vi "loopback cluster (in place).vi"() -> ()   [LabVIEW 2013]
uses:
  Source/Pipes/Classes/Unix Pipe Reader/Open Pipe (reader).vi
  Source/Pipes/Classes/Unix Pipe Writer/Open Pipe (writer).vi
  Source/Pipes/Classes/Unix Pipe Reader/Close Pipe (reader).vi
  Source/Pipes/Classes/Unix Pipe Writer/Close Pipe (writer).vi
  <vilib>/NI/NI Linux RT Utilities/VIs/Public/Time/Get Clock Time (timespec).vi
  <vilib>/NI/NI Linux RT Utilities/Linux RT Utilities.lvlib
  Source/Pipes/Linux RT IPC.Pipes.lvlib
  Source/Pipes/Classes/Unix Pipe Writer/Unix Pipe Writer.lvclass
  Source/Pipes/Classes/Unix Pipe Reader/Unix Pipe Reader.lvclass
panel:
  out "read iterations":i32
  out "write iterations":i32
  in  "write":bool
  out "timed out":bool
  out "stop":bool
  out "pipe already exists?":bool
  in  "stop":bool
  out "time":cluster{"sec":u64, "nsec":u64}
  out "bytes read":i32
  out "error out":errorcluster
  out "bytes written":i32
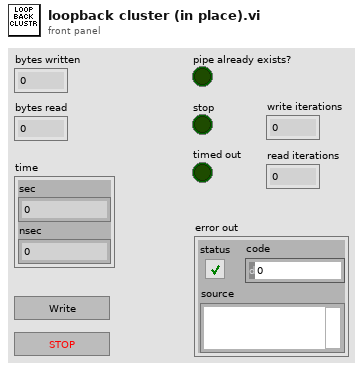
[diagram p1: front panel]
types:
  T1 = cluster{"Stop":bool, "Time":cluster{"sec":u64, "nsec":u64}}
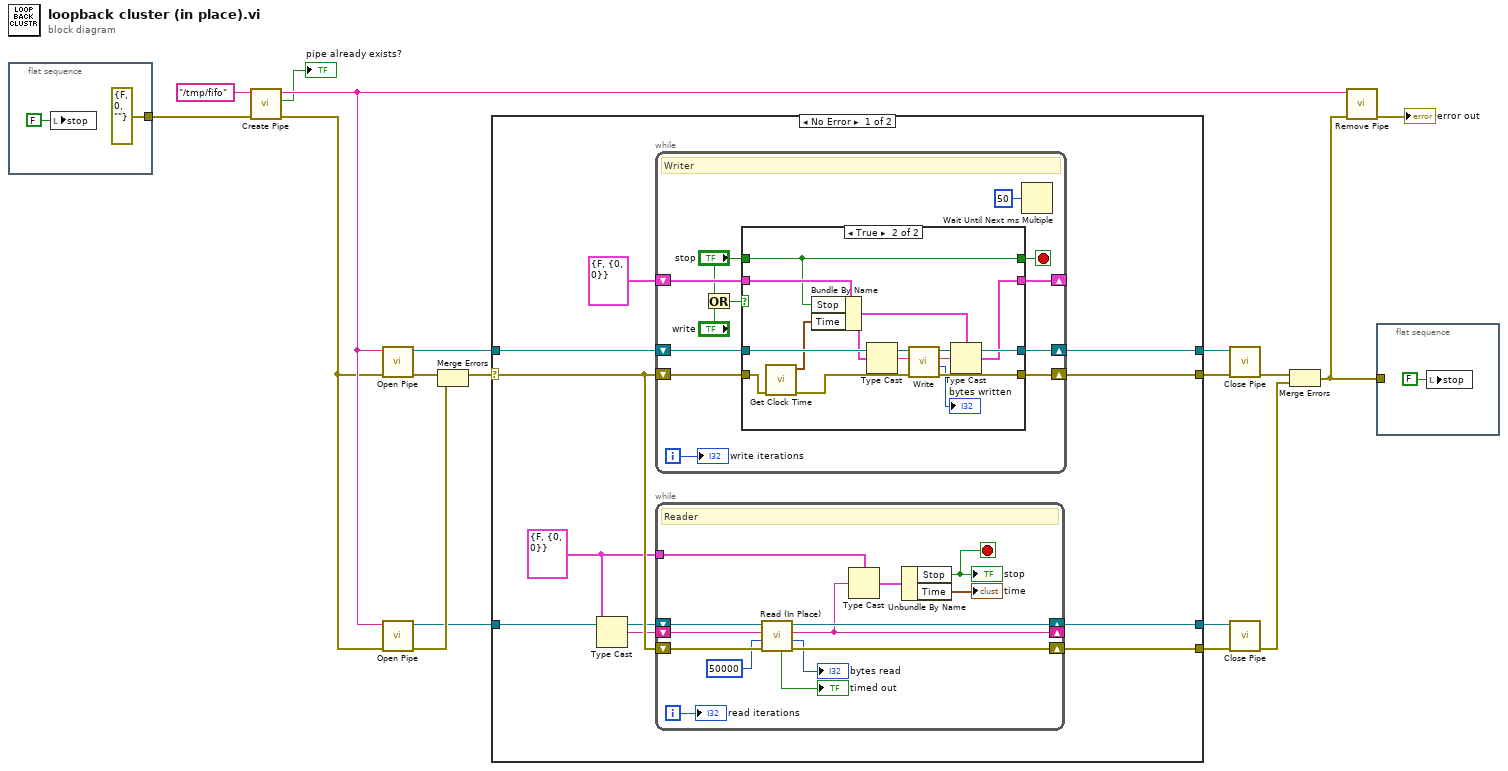
[diagram p0: block diagram]
diagram:
  n1 = flat-sequence {
    tunnel: [errorcluster {"status"=FALSE, "code"=0, "source"=""} ("error in (no error)")] -> w3
    frame #0 {
      n2 = local write "stop"(FALSE ("stop")) -> ()
    }
  }
  n3 = call "Create Pipe.vi"("error in (no error)"=w3, "pathname in"="/tmp/fifo") -> ("error out"=w1:errorcluster, "pipe already exists?"=→"pipe already exists?":bool, "pathname out"=w17:string)  [unwired: 7 in]
  n4 = call-poly "Open Pipe.vi"("error in (no error)"=w1, "pathname in"=w17) -> ("error out"=w7:errorcluster, "pipe writer out"=w14:refnum<data-value>)  [unwired: 8 in]
  n5 = call-poly "Open Pipe.vi"("error in (no error)"=w1, "pathname in"=w17) -> ("error out"=w6:errorcluster, "pipe reader out"=w4:refnum<data-value>)  [unwired: 8 in]
  n6 = Merge Errors(w7, w6) -> (w5:errorcluster)
  n7 = case shown="No Error" w5 {
    selector: w5 -> [w25 w74]
    tunnel: w14 -> [w30 w75]
    tunnel: [w29 w75] -> w13
    tunnel: [w28 w74] -> w12
    tunnel: w4 -> [w24 w73]
    tunnel: [w27 w73] -> w11
    tunnel: [w26 w74] -> w10
    frame No Error {
      w22 = T1 {"Stop"=FALSE, "Time"={"sec"=0, "nsec"=0}}
      n8 = Type Cast(x=w22) -> (*(type *) &x=w21:string)  [unwired: 1 in]
      n9 = while {
        shift-right: [w56] -> w29
        shift-left: w30 -> [w53]
        shift-right: [w55] -> w28
        shift-left: w25 -> [w52]
        shift-right: [w50] -> _
        shift-left: T1 {"Stop"=FALSE, "Time"={"sec"=0, "nsec"=0}} -> [w51]
        i -> [w54]
        stop <- w49 stop-if-true
        # "Writer"
        n10 = Or(x="stop", y="write") -> (x .or. y?=w45:bool)
        n11 = case shown="True" w45 {
          tunnel: [w58 w72] -> w56
          tunnel: [w57 w71] -> w55
          tunnel: w53 -> [w58 w70]
          tunnel: w52 -> [w57 w69]
          tunnel: w51 -> [w59 w67]
          tunnel: [w59 w61] -> w50
          tunnel: [_ w62] -> w49
          tunnel: "stop" -> [_ w62]
          frame False {
          }
          frame True {
            n12 = call-poly <vilib>:"Get Clock Time.vi"("error in (no error)"=w69) -> ("error out"=w68:errorcluster, "timespec"=w63:cluster{"sec":u64, "nsec":u64})  [unwired: 9 in]
            n13 = Bundle By Name(cluster=w67, "Stop"=w62, "Time"=w63) -> (w64:T1)
            n14 = Type Cast(x=w64) -> (*(type *) &x=w66:string)  [unwired: 1 in]
            n15 = call "Write.vi"("error in (no error)"=w68, "data"=w66, "pipe writer in"=w70) -> ("error out"=w71:errorcluster, "bytes written"=→"bytes written":i32, "data out"=w65:string, "pipe writer out"=w72:refnum<data-value>)  [unwired: 5 in]
            n16 = Type Cast(type=w64, x=w65) -> (*(type *) &x=w61:T1)
          }
        }
        n17 = Wait Until Next ms Multiple(millisecond multiple=u32 50) -> ()  [unwired: 1 out]
        "write iterations" <- w54
      }
      n18 = while {
        shift-right: [w42] -> w27
        shift-left: w24 -> [w44]
        shift-right: [w41] -> w26
        shift-left: w25 -> [w43]
        shift-right: [w31] -> _
        shift-left: w21 -> [w34]
        tunnel: w22 -> [w32]
        i -> [w39]
        stop <- w36 stop-if-true
        # "Reader"
        n19 = call "Read (In Place).vi"("error in (no error)"=w43, "timeout us (-1)"=i64 50000, "preallocated data in"=w34, "pipe reader in"=w44) -> ("error out"=w41:errorcluster, "bytes read"=→"bytes read":i32, "data out"=w31:string, "pipe reader out"=w42:refnum<data-value>, "timed out?"=→"timed out":bool)  [unwired: 3 in]
        n20 = Type Cast(type=w32, x=w31) -> (*(type *) &x=w33:T1)
        n21 = Unbundle By Name(w33) -> ("Stop"=w36:bool, "Time"=→"time":cluster{"sec":u64, "nsec":u64})
        "stop" <- w36
        "read iterations" <- w39
      }
    }
    frame Error {
    }
  }
  n22 = call-poly "Close Pipe.vi"("error in (no error)"=w12, "pipe in"=w13) -> ("error out"=w9:errorcluster)  [unwired: 8 in, 1 out]
  n23 = call-poly "Close Pipe.vi"("error in (no error)"=w10, "pipe in"=w11) -> ("error out"=w8:errorcluster)  [unwired: 8 in, 1 out]
  n24 = Merge Errors(w9, w8) -> (w2:errorcluster)
  n25 = call "Remove Pipe.vi"("error in (no error)"=w2, "pathname in"=w17) -> ("error out"=→"error out":errorcluster)  [unwired: 9 in]
  n26 = flat-sequence {
    tunnel: w2 -> [_]
    frame #0 {
      n27 = local write "stop"(FALSE ("stop")) -> ()
    }
  }
